vi "GetStringRef.vi"(0 "reference in":refnum<class "DataObject.lvclass">, 5 "error in (no error)":errorcluster) -> (14 "reference out":refnum<class "DataObject.lvclass">, 15 "StringRef":refnum<vi>, 19 "error out":errorcluster)   [LabVIEW 2020, in "DataObject.lvclass"]
uses:
  DataObject.lvclass
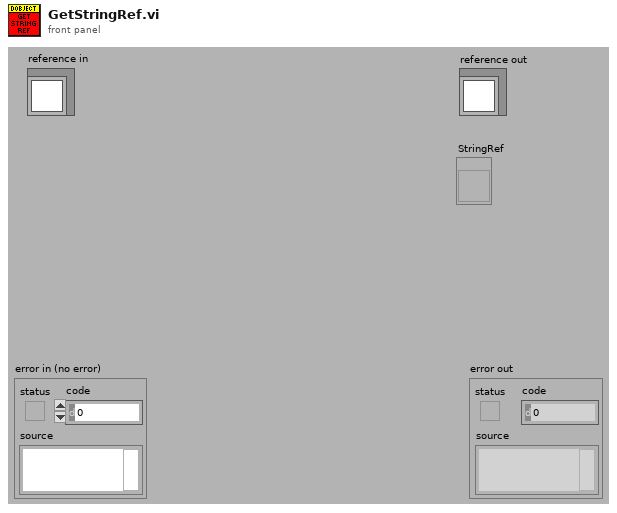
[diagram p1: front panel]
types:
  T1 = typedef "DataObject.lvclass/ObjectAttributes.ctl" = cluster{"StringRef":refnum<vi>}
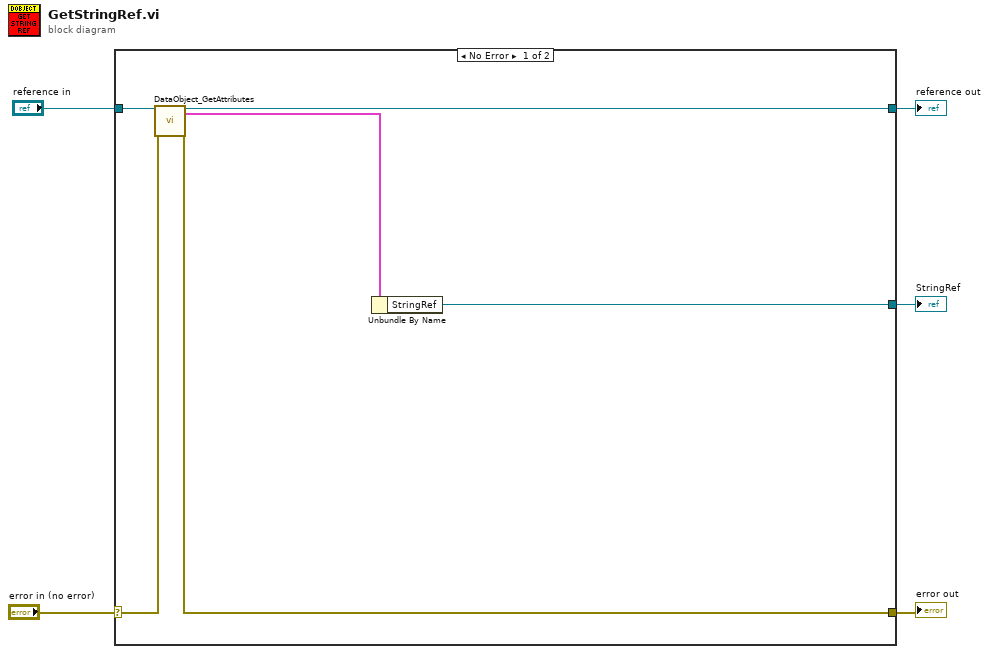
[diagram p0: block diagram]
diagram:
  n1 = case shown="No Error" "error in (no error)" {
    selector: "error in (no error)" -> [w11 w13]
    tunnel: [w9 w13] -> w4
    tunnel: [w7 w12] -> w2
    tunnel: "reference in" -> [w8 w12]
    tunnel: [w6 _] -> w1
    frame No Error {
      n2 = call "DataObject_GetAttributes.vi"("reference in"=w8, "error in (no error)"=w11) -> ("reference out"=w7:refnum<class "DataObject.lvclass">, "Data"=w10:T1, "error out"=w9:errorcluster)  [unwired: 14 in, 1 out]
      n3 = Unbundle By Name(w10) -> ("StringRef"=w6:refnum<vi>)
    }
    frame Error {
    }
  }
  "error out" <- w4
  "reference out" <- w2
  "StringRef" <- w1
